vi "Teleop.vi"(10 "Match Info":T2={"Autonomous Elapsed Seconds"=0.0, "TeleOp Elapsed Seconds"=0.0, "Disabled Elapsed Seconds"=0.0, "Visited Autonomous"=FALSE, "Visited TeleOp"=FALSE, "Visited Disabled"=FALSE, "Autonomous Settings"={"Autonomous Style"=enum."Independent", "VI Refnum"=refnum}}, 11 "Call Context":T3) -> ()   [LabVIEW 2014]
doc: "This VI is called for each TeleOp packet received from the DS where the robot is not disabled. It is often used to read from the joysticks and update I/O or to update setpoints for timed control loops. It should complete and return within 20 milliseconds or it may miss DS packets."
uses:
  <vilib>/Rock Robotics/Network Tables/SD Read Boolean.vi
  <vilib>/Rock Robotics/Network Tables/SD Read Number.vi
  <vilib>/Rock Robotics/WPI/Solenoid/WPI_SolenoidSetEnum.vi
  <vilib>/Rock Robotics/WPI/DriverStation/WPI_DriverStationMatch Info.ctl
  <vilib>/Rock Robotics/WPI/DriverStation/WPI_DriverStationDerivedRobotMode.ctl
  <vilib>/Rock Robotics/WPI/Solenoid/WPI_SolenoidValue.ctl
panel:
  in  "Solenoid 0":T1
  in  "Solenoid 3":T1
  in  "Solenoid 2":T1
  in  "Solenoid 1":T1
  out "Sample Slider 0":dbl(slide) scale=0.0..5.0
  out "Sample Boolean 1":bool
  out "Sample Boolean 0":bool
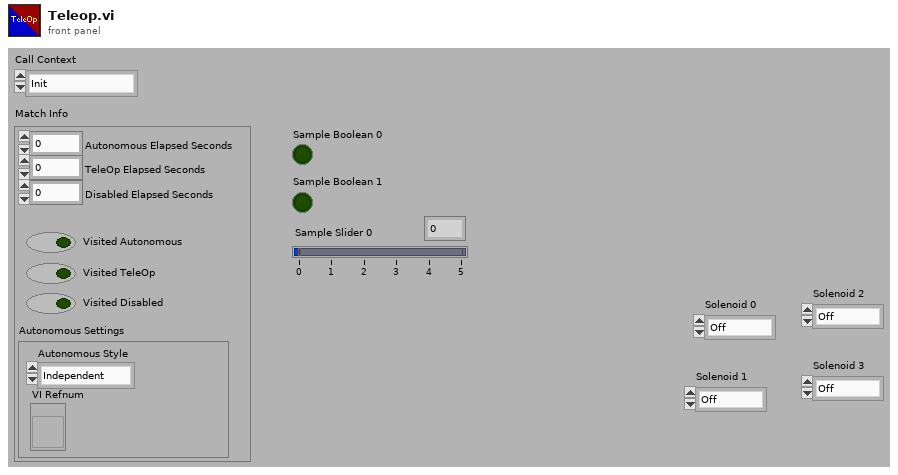
[diagram p1: front panel]
types:
  T1 = typedef "WPI_SolenoidValue.ctl" = enum16{"Off", "On", "Forward", "Reverse"}
  T2 = typedef "WPI_DriverStationMatch Info.ctl" = cluster{"Autonomous Elapsed Seconds":dbl, "TeleOp Elapsed Seconds":dbl, "Disabled Elapsed Seconds":dbl, "Visited Autonomous":bool, "Visited TeleOp":bool, "Visited Disabled":bool, "Autonomous Settings":cluster{"Autonomous Style":enum16{"Iterative", "Independent"}, "VI Refnum":refnum<vi>}}
  T3 = typedef "WPI_DriverStationDerivedRobotMode.ctl" = enum16{"Init", "Execute", "Stop"}
  T4 = typedef "WPI_JoystickDevRef.ctl" = cluster{"Device":T5}
  T5 = typedef "WPI_JoystickDeviceEnum.ctl" = enum16{"USB 0", "USB 1", "USB 2", "USB 3", "USB 4", "USB 5"}
  T6 = cluster{"Axes[0]":dbl, "Axes[1]":dbl, "Axes[2]":dbl, "Axes[3]":dbl, "Axes[4]":dbl, "Axes[5]":dbl, "Axes[6]":dbl, "Axes[7]":dbl, "Axes[8]":dbl}
  T7 = typedef "WPI_MotorControlDeviceRef.ctl" = cluster{"DeviceStatus":errorcluster, "Type":T8, "PWM":cluster{"Controller":T9, "PWM Channel":T10, "DeadBand":T11}, "CAN":cluster{"Device Number":u8, "Control Mode":T12, "Semaphore":T13, "Max Vout":dbl, "TalonSRX Control Mode":T14}, "Invert":bool, "TransformRef":T15, "InvTransformRef":T15}
  T8 = typedef "WPI_MotorControlType.ctl" = enum16{"PWM", "CAN", "CANTalonSRX"}
  T9 = typedef "FPGA_TypedefDigitalModule.ctl" = enum16{"Controller 1"}
  T10 = typedef "FPGA_DIOPWMChannel.ctl" = enum8{"PWM 0", "PWM 1", "PWM 2", "PWM 3", "PWM 4", "PWM 5", "PWM 6", "PWM 7", "PWM 8", "PWM 9", "PWM MXP 0", "PWM MXP 1", "PWM MXP 2", "PWM MXP 3", "PWM MXP 4", "PWM MXP 5", "PWM MXP 6", "PWM MXP 7", "PWM MXP 8", "PWM MXP 9", "Invalid"}
  T11 = typedef "WPI_PWMDeadband.ctl" = cluster{"Name":string, "maxPositivePwm":i32, "minPositivePwm":i32, "centerPwm":i32, "maxNegativePwm":i32, "minNegativePwm":i32, "angularRange":u16}
  T12 = typedef "WPI_CANJaguar_ControlMode.ctl" = enum8{"Percent VBus", "Current", "Speed", "Position", "Voltage"}
  T13 = typedef "Semaphore RefNum" = refnum<k1>
  T14 = typedef "WPI_CANTalonSRX_APIControlMode.ctl" = enum8{"Percent VBus", "Speed", "Position", "Slave", "Unchanged / Invalid"}
  T15 = typedef "WPI_PWMTransform_ConPane.ctl" = refnum<vi>
  T16 = cluster{"Buttons[0]":bool, "Buttons[1]":bool, "Buttons[2]":bool, "Buttons[3]":bool, "Buttons[4]":bool, "Buttons[5]":bool, "Buttons[6]":bool, "Buttons[7]":bool, "Buttons[8]":bool}
  T17 = typedef "WPI_SolenoidDevRef.ctl" = cluster{"DevStatus":errorcluster, "Pneumatics Control Module":u8, "Forward Solenoid Channel":T18, "Reverse Solenoid Channel":T18}
  T18 = typedef "WPI_SolenoidChannel.ctl" = enum8{"Solenoid 0", "Solenoid 1", "Solenoid 2", "Solenoid 3", "Solenoid 4", "Solenoid 5", "Solenoid 6", "Solenoid 7", "Invalid"}
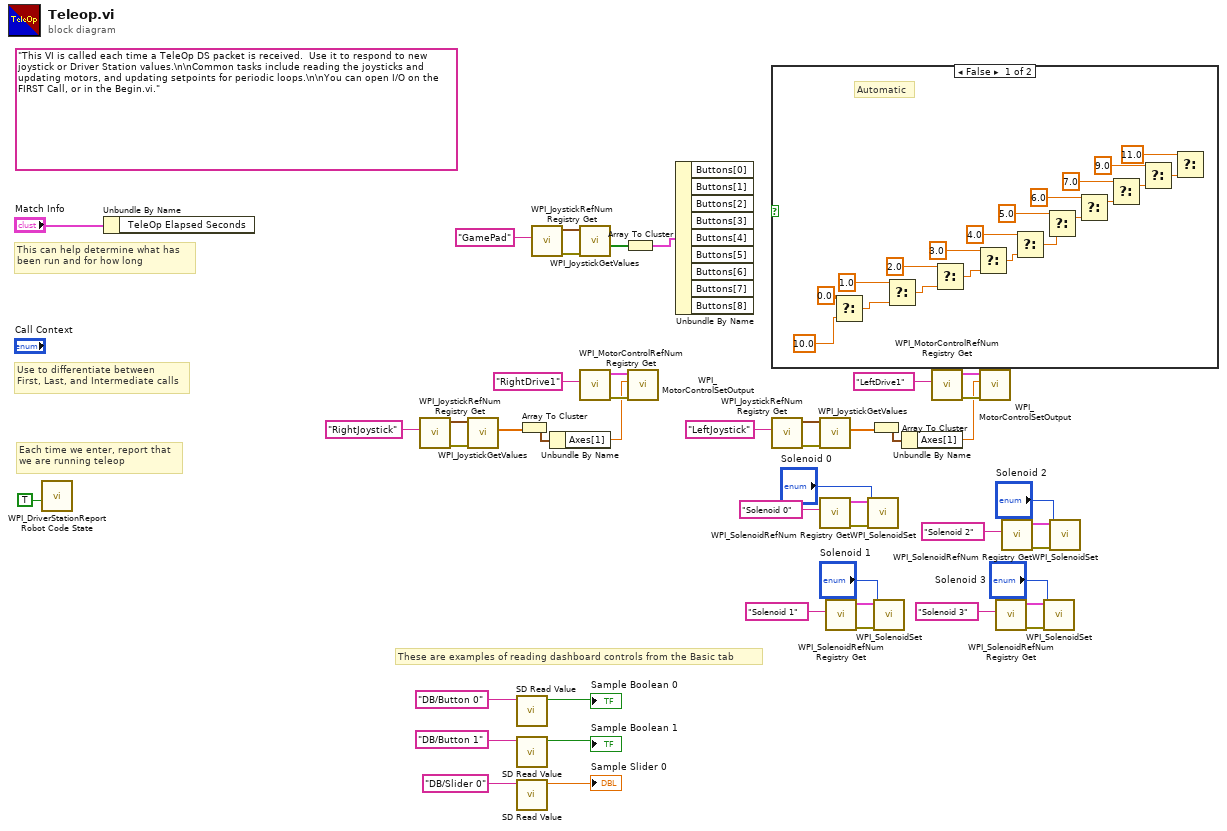
[diagram p0: block diagram]
diagram:
  (unwired) "This VI is called each time a TeleOp DS packet is received.  Use it to respond to new joystick or Driver Station values.\n\nCommon tasks include reading the joysticks and updating motors, and updating setpoints for periodic loops.\n\nYou can open I/O on the FIRST Call, or in the Begin.vi."
  # "These are examples of reading dashboard controls from the Basic tab"
  # "Each time we enter, report that\nwe are running teleop"
  # "Use to differentiate between\nFirst, Last, and Intermediate calls"
  # "This can help determine what has\nbeen run and for how long"
  n1 = call <vilib>:"WPI_DriverStationReport Robot Code State.vi"("TeleOp"=TRUE ("Autonomous")) -> ()  [unwired: 10 in, 1 out]
  n2 = Unbundle By Name("Match Info") -> ()  [unwired: 1 out]
  n3 = call <vilib>:"WPI_JoystickRefNum Registry Get.vi"("refnum name"="RightJoystick") -> ("error out"=w36:errorcluster, "JoystickDevRef"=w35:T4)  [unwired: 9 in]
  n4 = call <vilib>:"WPI_JoystickGetValues.vi"("error in (no error)"=w36, "JoystickDevRef"=w35) -> ("Axes"=w34:dbl[])  [unwired: 5 in, 4 out]
  n5 = call-poly <vilib>:"SD Read Value.vi"("Name"="DB/Button 0" ("refnum name")) -> ("Boolean"=→"Sample Boolean 0":bool)  [unwired: 8 in, 2 out]
  n6 = call-poly <vilib>:"SD Read Value.vi"("Name"="DB/Button 1" ("refnum name")) -> ("Boolean"=→"Sample Boolean 1":bool)  [unwired: 8 in, 2 out]
  n7 = call-poly <vilib>:"SD Read Value.vi"("Name"="DB/Slider 0" ("refnum name")) -> ("Numeric"=→"Sample Slider 0":dbl)  [unwired: 8 in, 2 out]
  n8 = Array To Cluster(array=w34) -> (cluster=w33:T6)
  n9 = call <vilib>:"WPI_JoystickRefNum Registry Get.vi"("refnum name"="GamePad") -> ("error out"=w9:errorcluster, "JoystickDevRef"=w8:T4)  [unwired: 9 in]
  n10 = Unbundle By Name(w33) -> ("Axes[1]"=w23:dbl)
  n11 = call <vilib>:"WPI_JoystickGetValues.vi"("error in (no error)"=w9, "JoystickDevRef"=w8) -> ("Buttons"=w6:bool[])  [unwired: 5 in, 4 out]
  n12 = call <vilib>:"WPI_MotorControlRefNum Registry Get.vi"("refnum name"="RightDrive1") -> ("error out"=w39:errorcluster, "MotorControlDevRef"=w38:T7)  [unwired: 9 in]
  n13 = Array To Cluster(array=w6) -> (cluster=w5:T16)
  n14 = call <vilib>:"WPI_MotorControlSetOutput.vi"("error in (no error)"=w39, "Output"=w23, "MotorControlDevRef"=w38) -> ()  [unwired: 6 in, 3 out]
  n15 = Unbundle By Name(w5) -> ()  [unwired: 9 out]
  n16 = case shown="False" {
    selector: _ -> [_ _]
    frame False {
      # "Automatic"
      n17 = Select(t=0.0, f=10.0) -> (s? t:f=w65:dbl)  [unwired: 1 in]
      n18 = Select(t=1.0, f=w65) -> (s? t:f=w63:dbl)  [unwired: 1 in]
      n19 = Select(t=2.0, f=w63) -> (s? t:f=w61:dbl)  [unwired: 1 in]
      n20 = Select(t=3.0, f=w61) -> (s? t:f=w59:dbl)  [unwired: 1 in]
      n21 = Select(t=4.0, f=w59) -> (s? t:f=w57:dbl)  [unwired: 1 in]
      n22 = Select(t=5.0, f=w57) -> (s? t:f=w55:dbl)  [unwired: 1 in]
      n23 = Select() -> ()  [unwired: 3 in, 1 out]
      n24 = Select(t=6.0, f=w55) -> (s? t:f=w53:dbl)  [unwired: 1 in]
      n25 = Select(t=7.0, f=w53) -> (s? t:f=w51:dbl)  [unwired: 1 in]
      n26 = Select(t=9.0, f=w51) -> (s? t:f=w49:dbl)  [unwired: 1 in]
      n27 = Select(t=11.0, f=w49) -> ()  [unwired: 1 in, 1 out]
    }
    frame True {
    }
  }
  n28 = call <vilib>:"WPI_JoystickRefNum Registry Get.vi"("refnum name"="LeftJoystick") -> ("error out"=w28:errorcluster, "JoystickDevRef"=w27:T4)  [unwired: 9 in]
  n29 = call <vilib>:"WPI_JoystickGetValues.vi"("error in (no error)"=w28, "JoystickDevRef"=w27) -> ("Axes"=w26:dbl[])  [unwired: 5 in, 4 out]
  n30 = call <vilib>:"WPI_SolenoidRefNum Registry Get.vi"("refnum name"="Solenoid 0") -> ("error out"=w4:errorcluster, "SolenoidDevRef"=w3:T17)  [unwired: 9 in]
  n31 = call <vilib>:"WPI_SolenoidRefNum Registry Get.vi"("refnum name"="Solenoid 1") -> ("error out"=w21:errorcluster, "SolenoidDevRef"=w20:T17)  [unwired: 9 in]
  n32 = call-poly <vilib>:"WPI_SolenoidSet.vi"("error in (no error)"=w4, "Value"="Solenoid 0", "SolenoidDevRef"=w3) -> ()  [unwired: 7 in, 2 out]
  n33 = Array To Cluster(array=w26) -> (cluster=w25:T6)
  n34 = call-poly <vilib>:"WPI_SolenoidSet.vi"("error in (no error)"=w21, "Value"="Solenoid 1", "SolenoidDevRef"=w20) -> ()  [unwired: 7 in, 2 out]
  n35 = Unbundle By Name(w25) -> ("Axes[1]"=w22:dbl)
  n36 = call <vilib>:"WPI_MotorControlRefNum Registry Get.vi"("refnum name"="LeftDrive1") -> ("error out"=w31:errorcluster, "MotorControlDevRef"=w30:T7)  [unwired: 9 in]
  n37 = call <vilib>:"WPI_MotorControlSetOutput.vi"("error in (no error)"=w31, "Output"=w22, "MotorControlDevRef"=w30) -> ()  [unwired: 6 in, 3 out]
  n38 = call <vilib>:"WPI_SolenoidRefNum Registry Get.vi"("refnum name"="Solenoid 3") -> ("error out"=w13:errorcluster, "SolenoidDevRef"=w12:T17)  [unwired: 9 in]
  n39 = call <vilib>:"WPI_SolenoidRefNum Registry Get.vi"("refnum name"="Solenoid 2") -> ("error out"=w17:errorcluster, "SolenoidDevRef"=w16:T17)  [unwired: 9 in]
  n40 = call-poly <vilib>:"WPI_SolenoidSet.vi"("error in (no error)"=w13, "Value"="Solenoid 3", "SolenoidDevRef"=w12) -> ()  [unwired: 7 in, 2 out]
  n41 = call-poly <vilib>:"WPI_SolenoidSet.vi"("error in (no error)"=w17, "Value"="Solenoid 2", "SolenoidDevRef"=w16) -> ()  [unwired: 7 in, 2 out]
